vi "Configure List Operation.vi"(0 "VISA resource name":refnum<visa-resource-name>, 5 "Range (15)":dbl=15.0001 min=0.0001 max=240.0 step=1.0 format="%.2g", 7 "List Count (1)":i32=1 min=1 max=65536 step=1 format="%.0g", 9 "Total Steps (2)":i32=2 min=2 max=84 step=1 format="%.0g", 11 "error in (no error)":errorcluster, 12 "Rate (0:High)":u16(ring) items=["High", "Low"]) -> (4 "VISA resource name out":refnum<visa-resource-name>, 15 "error out":errorcluster)   [LabVIEW 2018, in "BK Precision 8600 Series.lvlib"]
doc: "Configures parameters for list mode operation. This VI should be used to setup the list before running <b>Configure List Step Parameters.vi</b>.\n\nNote: List mode is only available for CC mode."
uses:
  <instrlib>/BK Precision 8600 Series/BK Precision 8600 Series.lvlib
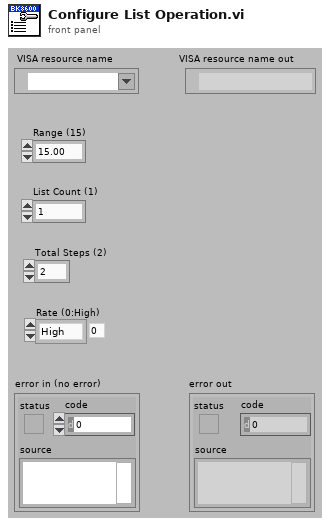
[diagram p1: front panel]
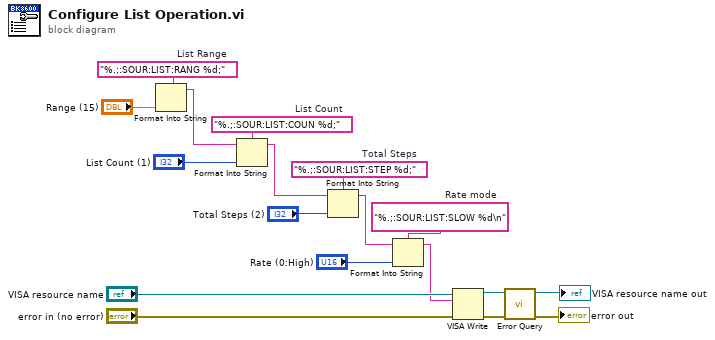
[diagram p0: block diagram]
diagram:
  w4 = "%.;:SOUR:LIST:SLOW %d\n"  # Rate mode
  w9 = "%.;:SOUR:LIST:STEP %d;"  # Total Steps
  w12 = "%.;:SOUR:LIST:COUN %d;"  # List Count
  w14 = "%.;:SOUR:LIST:RANG %d;"  # List Range
  n1 = Format Into String(format string=w14, "Range (15)") -> (resulting string=w10:string)  [unwired: 2 in, 1 out]
  n2 = Format Into String(format string=w12, initial string=w10, "List Count (1)") -> (resulting string=w5:string)  [unwired: 1 in, 1 out]
  n3 = Format Into String(format string=w9, initial string=w5, "Total Steps (2)") -> (resulting string=w2:string)  [unwired: 1 in, 1 out]
  n4 = Format Into String(format string=w4, initial string=w2, "Rate (0:High)") -> (resulting string=w1:string)  [unwired: 1 in, 1 out]
  n5 = VISA Write(VISA resource name="VISA resource name", write buffer=w1, error in (no error)="error in (no error)") -> (VISA resource name out=w17:refnum<visa-resource-name>, error out=w18:errorcluster)  [unwired: 1 out]
  n6 = call <instrlib>:"Error Query.vi"("error in (no error)"=w18, "VISA resource name"=w17) -> ("error out"=→"error out":errorcluster, "VISA resource name out"=→"VISA resource name out":refnum<visa-resource-name>)  [unwired: 6 in, 2 out]
